vi "New Server Thread.vi"(1 "connection ID":refnum<k5>) -> (0 "Server Thread":T1)   [LabVIEW 2016]
uses:
  Server Thread.ctl
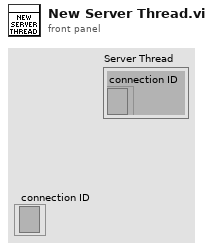
[diagram p1: front panel]
types:
  T1 = typedef "Server Thread.ctl" = cluster{"connection ID":refnum<k5>}
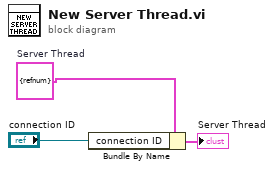
[diagram p0: block diagram]
diagram:
  w2 = T1 {"connection ID"=refnum}  # Server Thread
  n1 = Bundle By Name(cluster=w2, "connection ID"="connection ID") -> (→"Server Thread":T1)
